vi "Clear Scan Time Out_test.vi"(7 "ESP32 ref":refnum<visa-resource-name>="COM4", 8 "error in (no error)":errorcluster, 11 "VISA Refnum in":refnum<visa-resource-name>) -> (0 "error out":errorcluster, 1 "error?":bool, 2 "Time out count":i32, 3 "VISA Refnum out":refnum<visa-resource-name>, 4 "error in (no error) 2":errorcluster[](array[cluster]), 5 "ESP32 ref out":refnum<visa-resource-name>)   [LabVIEW 2023]
uses:
  <vilib>/Utility/error.llb/DialogType.ctl
panel:
  out "Measurements 3":dbl[](array[numeric])
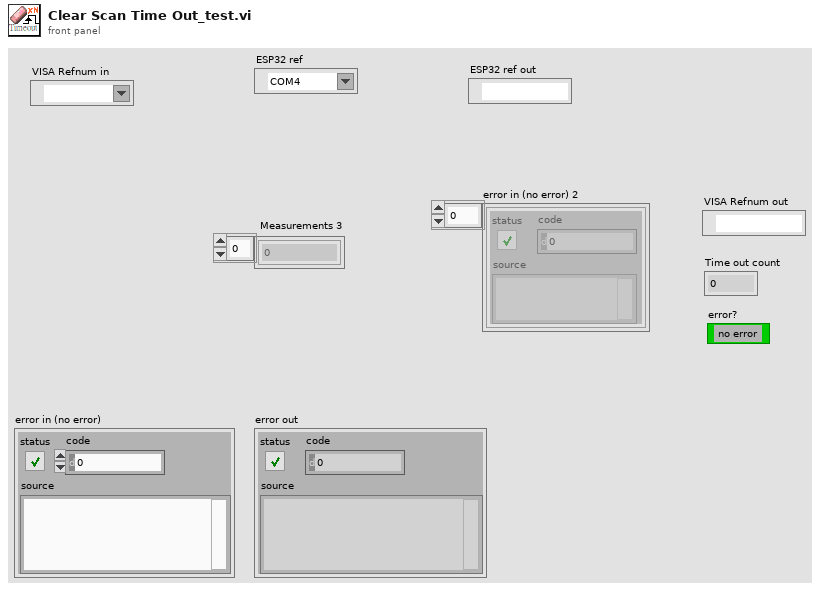
[diagram p1: front panel]
types:
  T1 = typedef "DialogType.ctl" = u16
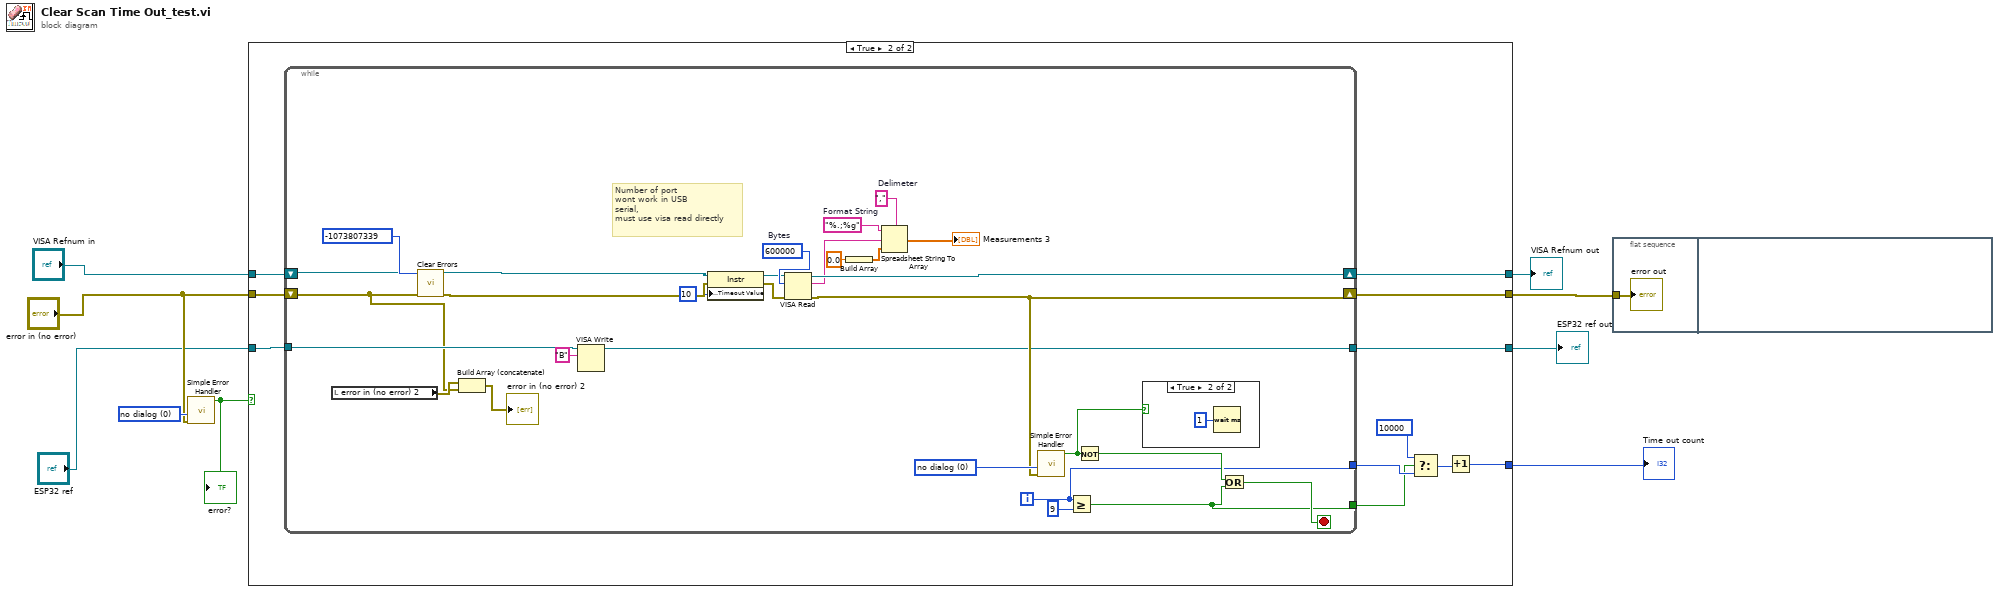
[diagram p0: block diagram]
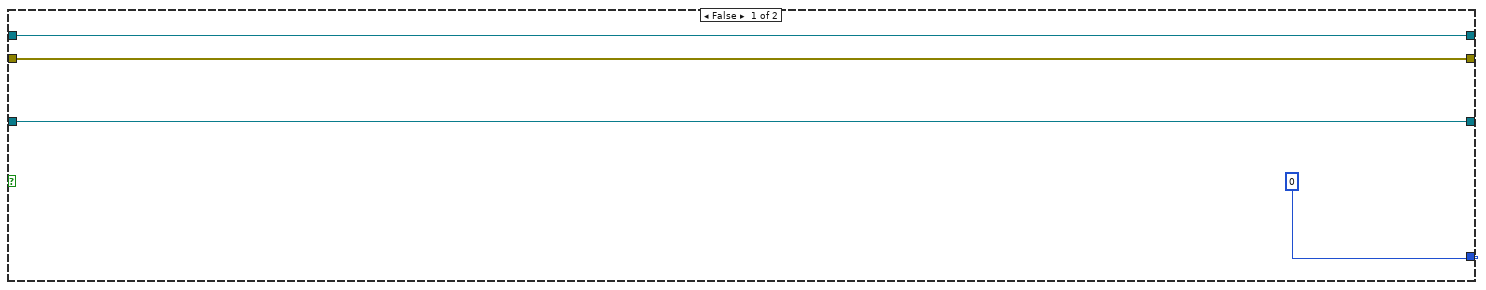
[diagram p2: hidden frame]
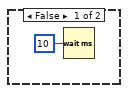
[diagram p3: hidden frame]
diagram:
  w6 = T1 0 items=["no dialog", "OK message", "continue or stop message", "OK message + warnings", "continue/stop + warnings"] ("type of dialog (OK msg:1)")
  n1 = call <vilib>:"Simple Error Handler.vi"("type of dialog (OK msg:1)"=w6, "error in (no error)"="error in (no error)") -> ("error?"=w4:bool)  [unwired: 3 in, 4 out]
  "error?" <- w4
  n2 = case shown="True" w4 {
    tunnel: [w13 w24] -> w9
    tunnel: "error in (no error)" -> [w12 w23]
    tunnel: "VISA Refnum in" -> [w13 w22]
    tunnel: [w12 w21] -> w7
    tunnel: [0 w20] -> w3
    tunnel: "ESP32 ref" -> [w10 w15]
    tunnel: [w10 w14] -> w1
    frame False {
    }
    frame True {
      n3 = while {
        shift-right: [w48] -> w21
        shift-left: w23 -> [w25]
        shift-right: [w52] -> w24
        shift-left: w22 -> [w30]
        tunnel: [w44] -> w18
        tunnel: [w43] -> w17
        tunnel: w15 -> [w29]
        tunnel: [w28] -> w14
        i -> [w44]
        stop <- w45 stop-if-true
        w39 = ","  # Delimeter
        w40 = "%.;%g"  # Format String
        w34 = u32 600000  # Bytes
        w49 = T1 0 items=["no dialog", "OK message", "continue or stop message", "OK message + warnings", "continue/stop + warnings"] ("type of dialog (OK msg:1)")
        # "Number of port\nwont work in USB \nserial,\nmust use visa read directly"
        n4 = local read "error in (no error) 2"() -> (w26:errorcluster[])
        n5 = call <vilib>:"Clear Errors.vi"("error in (no error)"=w25, "specific error code to clear (0: all)"=-1073807339 ("code out")) -> ("error out"=w50:errorcluster)  [unwired: 4 in, 1 out]
        n6 = Build Array (concatenate)(w26, w25) -> (→"error in (no error) 2":errorcluster[])
        n7 = VISA Write(VISA resource name=w29, write buffer="B") -> (VISA resource name out=w28:refnum<visa-resource-name>)  [unwired: 1 in, 2 out]
        n8 = property class="Instr"(reference=w30, error in=w50, "General Settings:Timeout Value"=u32 10) -> (reference out=w33:refnum<visa-resource-name>, error out=w32:errorcluster)
        n9 = VISA Read(VISA resource name=w33, byte count=w34, error in (no error)=w32) -> (VISA resource name out=w52:refnum<visa-resource-name>, read buffer=w35:string, error out=w48:errorcluster)  [unwired: 1 out]
        n10 = Build Array(0.0) -> (w37:dbl[])
        n11 = Spreadsheet String To Array(delimiter (Tab)=w39, format string=w40, spreadsheet string=w35, array type (2D Dbl)=w37) -> (array=→"Measurements 3":dbl[])
        n12 = call <vilib>:"Simple Error Handler.vi"("type of dialog (OK msg:1)"=w49, "error in (no error)"=w48) -> ("error?"=w42:bool)  [unwired: 3 in, 4 out]
        n13 = Greater Or Equal?(x=w44, y=9) -> (x >= y?=w43:bool)
        n14 = Not(x=w42) -> (.not. x?=w46:bool)
        n15 = case shown="True" w42 {
          frame False {
            n16 = Wait (ms)(milliseconds to wait=u32 10) -> ()  [unwired: 1 out]
          }
          frame True {
            n17 = Wait (ms)(milliseconds to wait=u32 1) -> ()  [unwired: 1 out]
          }
        }
        n18 = Or(x=w46, y=w43) -> (x .or. y?=w45:bool)
      }
      n19 = Select(t=10000, s=w17, f=w18) -> (s? t:f=w19:i32)
      n20 = Increment(x=w19) -> (x+1=w20:i32)
    }
  }
  "VISA Refnum out" <- w9
  "Time out count" <- w3
  "ESP32 ref out" <- w1
  n21 = flat-sequence {
    tunnel: w7 -> [w55]
    frame #0 {
      "error out" <- w55
    }
    frame #1 {
    }
  }
